vi "Launcher.vi"   [LabVIEW 2020]
uses:
  Application Manager/Application Manager/Application Manager.lvclass
  C:/Program Files/National Instruments/LabVIEW 2026/vi.lib/ActorFramework/Actor/Actor.lvclass
  <vilib>/Natan Biesmans/G2CPU GPU and CPU HPC Toolkit/G2CPU Libraries/Runtime Licensing/G2CPU License Check.vi
  <resource>/Natan Biesmans/G2CPU GPU and CPU HPC Toolkit/Garbage Collector/G2CPU GarbageCollectorFGV.vi
  <vilib>/Natan Biesmans/G2CPU GPU and CPU HPC Toolkit/G2CPU Libraries/Arrays/SubVI/G2CPU State.vi
  <vilib>/NI License Manager/Open Session.vi
  <vilib>/NI License Manager/Check License Status.vi
  <vilib>/NI License Manager/Check License Status (Single).vi
  <vilib>/NI License Manager/Activate License.vi
  <vilib>/NI License Manager/Activate License (Single).vi
  <vilib>/NI License Manager/Close Session.vi
  <vilib>/Natan Biesmans/G2CPU GPU and CPU HPC Toolkit/ArrayFire Driver/VIs/init.vi
  <vilib>/Natan Biesmans/G2CPU GPU and CPU HPC Toolkit/G2CPU Libraries/Async IO/CUDA Context FGV.vi
  <resource>/Natan Biesmans/G2CPU GPU and CPU HPC Toolkit/Garbage Collector/G2CPU DMAGarbageCollectorFGV.vi
  <vilib>/Natan Biesmans/G2CPU GPU and CPU HPC Toolkit/G2CPU Libraries/Arrays/Array/Array Prototype.lvclass
  <vilib>/ActorFramework/Actor/Actor.lvclass
  <vilib>/MGI/Monitored Actor/Monitored Actor.lvlib
panel:
  # "Loading the demo, please wait ..."
types:
  T1 = enum32{"Invalid", "Standard", "Closed", "Hidden", "Minimized", "Maximized"}
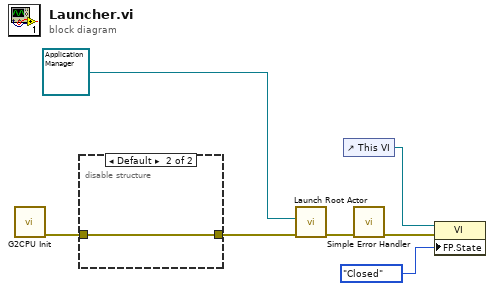
[diagram p0: block diagram]
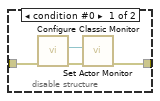
[diagram p2: hidden frame]
diagram:
  n1 = call <vilib>:"G2CPU Init.vi"() -> ("error out"=w1:errorcluster)  [unwired: 11 in]
  n2 = disable-structure shown="Default" {
    disable-tunnel: [w9 w12] -> w5
    disable-tunnel: w1 -> [w8 w12]
    frame condition #0 {
      n3 = call <vilib>:"Configure Classic Monitor.vi"("error in (no error)"=w8) -> ("error out"=w10:errorcluster, "Classic Monitor out"=w11:refnum<class "Actor Monitor.lvclass">)  [unwired: 9 in]
      n4 = call <vilib>:"Set Actor Monitor.vi"("error in (no error)"=w10, "Actor Monitor"=w11) -> ("error out"=w9:errorcluster)  [unwired: 9 in]
    }
    frame condition #1 (active) {
    }
  }
  n5 = call <vilib>:"Launch Root Actor.vi"("error in (no error)"=w5, "Actor"=refnum<class "Application Manager.lvclass"> refnum ("Application Manager.lvlib:Application Manager.lvclass")) -> ("error out"=w7:errorcluster)  [unwired: 8 in, 1 out]
  n6 = control-ref of="This VI"() -> (w3:refnum<vi>)
  n7 = call <vilib>:"Simple Error Handler.vi"("error in (no error)"=w7) -> ("error out"=w4:errorcluster)  [unwired: 4 in, 4 out]
  n8 = property class="VI"(reference=w3, error in=w4, "FP.State"=T1."Closed" ("Front Panel Window:State")) -> ()  [unwired: 2 out]
